vi "PropagateBeamNumeric.vi"(1 "q in":cluster{"qx":cdb, "qy":cdb}, 2 "Matrix":dbl[][](array[numeric])) -> (0 "q out":cluster{"qx":cdb, "qy":cdb})   [LabVIEW 2011]
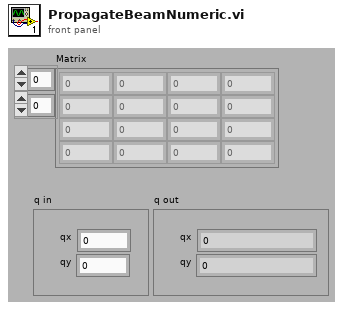
[diagram p1: front panel]
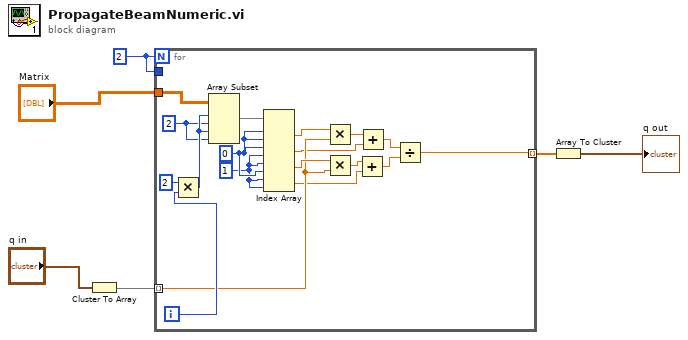
[diagram p0: block diagram]
diagram:
  w2 = 2
  n1 = Cluster To Array(cluster="q in") -> (array=w5:cdb[])
  n2 = for {
    N: w2 -> [_]
    tunnel: w5 -> [w14] mode=indexing
    tunnel: "Matrix" -> [w24]
    tunnel: [w7] -> w3 mode=indexing
    tunnel: w2 -> [_]
    i -> [w20]
    w17 = 1 ("dimension size")
    w18 = 0 ("dimension size")
    w21 = 2 ("length")
    n3 = Multiply(x=2, y=w20) -> (x*y=w22:i32)
    n4 = Array Subset(array=w24, index (row)=w22, length (row)=w21, index (col)=w22, length (col)=w21) -> (w19:dbl[][])
    n5 = Index Array(array=w19, index (row) #1=w18, index (col) #1=w18, index (row) #2=w18, index (col) #2=w17, index (row) #3=w17, index (col) #3=w18, index (row) #4=w17, index (col) #4=w17) -> (element #1=w16:dbl, element #2=w12:dbl, element #3=w15:dbl, element #4=w10:dbl)
    n6 = Multiply(x=w16, y=w14) -> (x*y=w13:cdb)
    n7 = Multiply(x=w15, y=w14) -> (x*y=w11:cdb)
    n8 = Add(x=w11, y=w10) -> (x+y=w8:cdb)
    n9 = Add(x=w13, y=w12) -> (x+y=w9:cdb)
    n10 = Divide(x=w9, y=w8) -> (x/y=w7:cdb)
  }
  n11 = Array To Cluster(array=w3) -> (cluster=→"q out":cluster{"[0]":cdb, "[1]":cdb})
